vi "Configure Noise Level.vi"(8 "error in":errorcluster, 10 "level":dbl, 11 "lia host in":refnum<class "LIA Host Interface RT.lvclass">) -> (0 "error out":errorcluster, 3 "lia host out":refnum<class "LIA Host Interface RT.lvclass">)   [LabVIEW 2018, in "LIA Host Interface RT.lvclass"]
uses:
  LIA Host Interface RT.lvclass
  shared/Public/message.ctl
  shared/Lock-In Amplifier Example Shared.lvlib
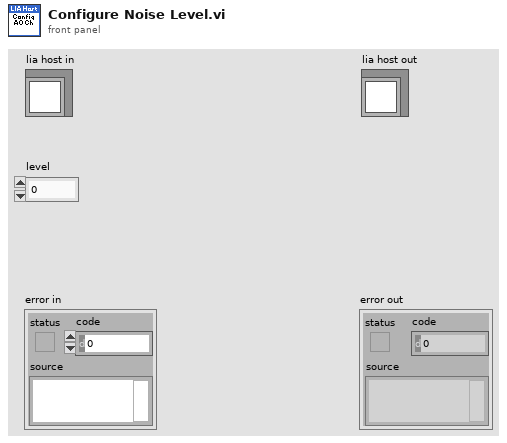
[diagram p1: front panel]
types:
  T1 = typedef "Lock-In Amplifier Example Shared.lvlib/message.ctl" = cluster{"command":u32, "payload":string}
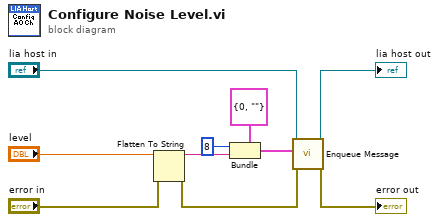
[diagram p0: block diagram]
diagram:
  n1 = Flatten To String(anything="level", error in (no error)="error in") -> (data string=w9:string, error out=w6:errorcluster)  [unwired: 2 in, 1 out]
  n2 = Bundle(cluster=T1 {"command"=0, "payload"=""} ("message"), "command"=u32 8, "payload"=w9) -> (w8:T1)
  n3 = call "Enqueue Message.vi"("error in"=w6, "command"=w8, "lia host in"="lia host in") -> ("error out"=→"error out":errorcluster, "lia host out"=→"lia host out":refnum<class "LIA Host Interface RT.lvclass">)  [unwired: 7 in]
